vi "CreateMoveAngle.vi"(6 "步进2":i32, 7 "步进1":i32, 8 "终止2":i32, 9 "起始2":i32, 10 "终止1":i32, 11 "起始1":i32) -> (3 "数组":i32[](array[numeric]))   [LabVIEW 2024]
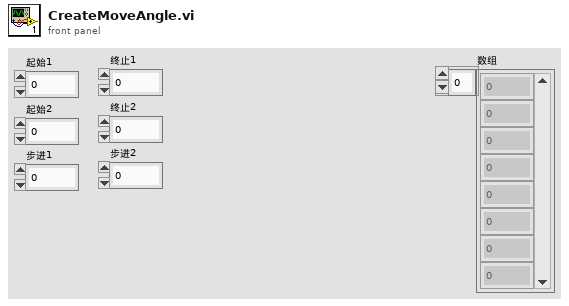
[diagram p1: front panel]
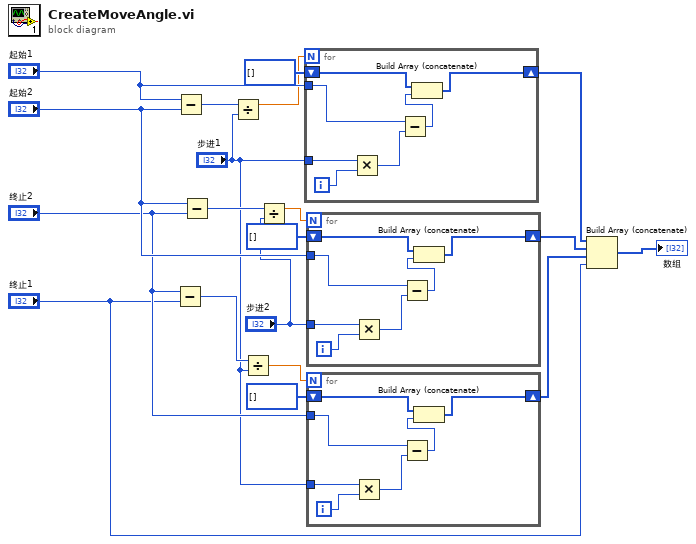
[diagram p0: block diagram]
diagram:
  n1 = Subtract(x="终止2", y="终止1") -> (x-y=w4:i32)
  n2 = Subtract(x="起始1", y="起始2") -> (x-y=w18:i32)
  n3 = Subtract(x="起始2", y="终止2") -> (x-y=w10:i32)
  n4 = Divide(x=w18, y="步进1") -> (x/y=w5:dbl)
  n5 = Divide(x=w4, y="步进1") -> (x/y=w2:dbl)
  n6 = Divide(x=w10, y="步进2") -> (x/y=w7:dbl)
  n7 = for {
    N: w5 -> [_]
    tunnel: "步进1" -> [w25]
    tunnel: "起始1" -> [w23]
    shift-right: [w21] -> w14
    shift-left: i32[] [] -> [w20]
    i -> [w26]
    n8 = Multiply(x=w25, y=w26) -> (x*y=w24:i32)
    n9 = Subtract(x=w23, y=w24) -> (x-y=w22:i32)
    n10 = Build Array (concatenate)(w20, w22) -> (w21:i32[])
  }
  n11 = for {
    N: w7 -> [_]
    tunnel: "步进2" -> [w32]
    tunnel: "起始2" -> [w30]
    shift-right: [w28] -> w13
    shift-left: i32[] [] -> [w27]
    i -> [w33]
    n12 = Multiply(x=w32, y=w33) -> (x*y=w31:i32)
    n13 = Subtract(x=w30, y=w31) -> (x-y=w29:i32)
    n14 = Build Array (concatenate)(w27, w29) -> (w28:i32[])
  }
  n15 = for {
    N: w2 -> [_]
    tunnel: "步进1" -> [w39]
    tunnel: "终止2" -> [w37]
    shift-right: [w35] -> w12
    shift-left: i32[] [] -> [w34]
    i -> [w40]
    n16 = Multiply(x=w39, y=w40) -> (x*y=w38:i32)
    n17 = Subtract(x=w37, y=w38) -> (x-y=w36:i32)
    n18 = Build Array (concatenate)(w34, w36) -> (w35:i32[])
  }
  n19 = Build Array (concatenate)(w14, w13, w12, "终止1") -> (→"数组":i32[])
